vi "JSON to LVObject - U16 Member - Should Parse Value.vi"() -> ()   [LabVIEW 2017, in "Generic Object Serializer Tests.lvlib"]
uses:
  Generic Object Serializer Tests.lvlib
  Generic Object Serializer/Generic Object Serializer.lvclass
  Numeric Types/Numeric Types.lvclass
  Generic Object Serializer/Type Name Handling.ctl
  Generic Object Serializer/Generic Object Serializer.lvclass/Generic Object Serializer.ctl
  Numeric Types/Numeric Types.lvclass/Numeric Types.ctl
  Generic Object Serializer/Write Type Name Handling.vi
  Numeric Types/Read U16.vi
  <vilib>/addons/_JKI Toolkits/Caraya/classes/Assert/Assert Equal Value_Variant.vi
  <vilib>/addons/_JKI Toolkits/Caraya/classes/Test/Test.lvclass
  <vilib>/addons/_JKI Toolkits/Caraya/classes/Assert/Assert.lvclass
panel:
  out "error out":errorcluster
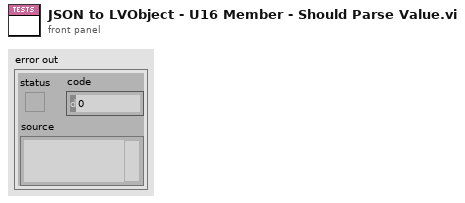
[diagram p1: front panel]
types:
  T1 = typedef "Generic Object Serializer.lvclass/Type Name Handling.ctl" = enum16{"None", "Inline"}
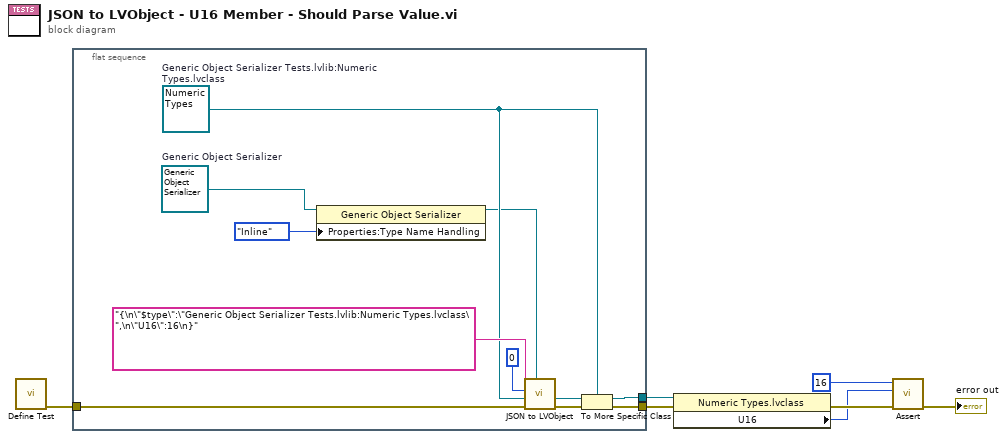
[diagram p0: block diagram]
diagram:
  n1 = call <vilib>:"Define Test.vi"() -> ("error out"=w7:errorcluster)  [unwired: 11 in]
  n2 = flat-sequence {
    tunnel: w7 -> [w9]
    tunnel: [w14] -> w3
    tunnel: [w8] -> w5
    frame #0 {
      w13 = refnum<class "Numeric Types.lvclass"> refnum  # Generic Object Serializer Tests.lvlib:Numeric Types.lvclass
      w18 = refnum<class "Generic Object Serializer.lvclass"> refnum  # Generic Object Serializer
      n3 = property class="Generic Object Serializer"(reference=w18, "Properties:Type Name Handling"=Type_Name_Handling."Inline" ("Type Name Handling")) -> (reference out=w11:refnum<class "Generic Object Serializer.lvclass">)  [unwired: 1 in, 1 out]
      n4 = call-dynamic "JSON to LVObject.vi"("LVClass Serializer"=w11, "error in (no error)"=w9, "Object Type"=w13, "Offset"=0, "JSON"="{\n\"$type\":\"Generic Object Serializer Tests.lvlib:Numeric Types.lvclass\",\n\"U16\":16\n}") -> ("error out"=w17:errorcluster, "Object"=w15:refnum<class>)  [unwired: 5 in]
      n5 = To More Specific Class(target class=w13, reference=w15, error in=w17) -> (specific class reference=w14:refnum<class "Numeric Types.lvclass">, error out=w8:errorcluster)
    }
  }
  n6 = property class="Numeric Types.lvclass"(reference=w3, error in=w5) -> (error out=w4:errorcluster, "U16"=w2:u16)  [unwired: 1 out]
  n7 = call-poly <vilib>:"Assert.vi"("error in (no error)"=w4, "Y"=w2, "X"=u16 16 ("Enum U8")) -> ("error out"=→"error out":errorcluster)  [unwired: 8 in]
